vi "Set CAN Adapter Names.vi"(10 "ICommunicate Names":string[](array[string]), 11 "Home in":refnum<class "Home.lvclass">) -> (3 "Home out":refnum<class "Home.lvclass">)   [LabVIEW 2020, in "Home.lvlib" / "Home.lvclass"]
uses:
  Home.lvclass
  Home.lvclass/Home.ctl
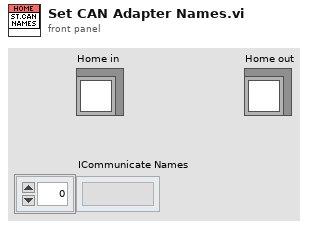
[diagram p1: front panel]
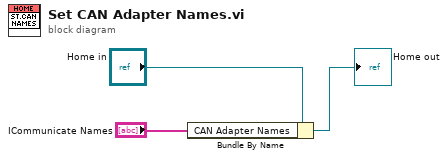
[diagram p0: block diagram]
diagram:
  n1 = Bundle By Name(cluster="Home in", "CAN Adapter Names"="ICommunicate Names") -> (→"Home out":refnum<class "Home.lvclass">)
